vi "PicoScope4000aExampleStreaming without queue220623.vi"() -> ()   [LabVIEW 2024]
uses:
  Global variables/Global 1.vi
  Global variables/filepath global variable.vi
  Global variables/global for picoscope.vi
  LabVIEW3D/PicoScope/Pico Technology/SDK/lib/ps4000a.dll
panel:
  out "result 2":dbl
  out "size (in bytes)":i64
  out "sampling period [s]":dbl=4.0000000000000003e-07
  in  ".pico filepath":path=path "F:/20240321-194116tdTomato/waveforms.pico"
  out "result":bool=TRUE
  out "record":bool=TRUE
  in  "start":bool
  in  "Channel settings":T1={"Ch D  sync"={"Enabled"=FALSE, "Coupling"=1, "Range"=7, "Offset"=0.0}, "Ch C AWG "={"Enabled"=TRUE, "Coupling"=1, "Range"=6, "Offset"=0.0}, "Ch G scape"={"Enabled"=TRUE, "Coupling"=1, "Range"=5, " Offset"=0.0}, "Ch H img scan"={"Enabled"=TRUE, "Coupling"=1, "Range"=7, "Offset"=0.0}, "Ch B Cam"={"Enabled"=TRUE, "Coupling"=1, "Range"=9, "Offset"=0.0}, "Ch A"={"Enabled"=FALSE, "Coupling"=1, "Range"=9, "Offset"=0.0}, "Ch E"={"Enabled"=FALSE, "Coupling"=1, "Range"=2, "Offset"=0.0}, "Ch F"={"Enabled"=FALSE, "Coupling"=1, "Range"=9, "Offset"=0.0}} {"Ch F"."Range" items=["10 mV", "20 mV", "50 mV", "100 mV", "200 mV", "500 mV", "1 V", "2 V", "5 V", "10 V", "20 V", "50 V ", "100 V"]; "Ch F"."Coupling" items=["AC", "DC"]; "Ch E"."Range" items=["10 mV", "20 mV", "50 mV", "100 mV", "200 mV", "500 mV", "1 V", "2 V", "5 V", "10 V", "20 V", "50 V ", "100 V"]; "Ch E"."Coupling" items=["AC", "DC"]; "Ch A"."Range" items=["10 mV", "20 mV", "50 mV", "100 mV", "200 mV", "500 mV", "1 V", "2 V", "5 V", "10 V", "20 V", "50 V ", "100 V"]; "Ch A"."Coupling" items=["AC", "DC"]; "Ch B Cam"."Range" items=["10 mV", "20 mV", "50 mV", "100 mV", "200 mV", "500 mV", "1 V", "2 V", "5 V", "10 V", "20 V", "50 V ", "100 V"]; "Ch B Cam"."Coupling" items=["AC", "DC"]; "Ch H img scan"."Range" items=["10 mV", "20 mV", "50 mV", "100 mV", "200 mV", "500 mV", "1 V", "2 V", "5 V", "10 V", "20 V", "50 V ", "100 V"]; "Ch H img scan"."Coupling" items=["AC", "DC"]; "Ch G scape"."Range" items=["10 mV", "20 mV", "50 mV", "100 mV", "200 mV", "500 mV", "1 V", "2 V", "5 V", "10 V", "20 V", "50 V ", "100 V"]; "Ch G scape"."Coupling" items=["AC", "DC"]; "Ch C AWG"."Range" items=["10 mV", "20 mV", "50 mV", "100 mV", "200 mV", "500 mV", "1 V", "2 V", "5 V", "10 V", "20 V", "50 V ", "100 V"]; "Ch C AWG"."Coupling" items=["AC", "DC"]; "Ch D  sync"."Range" items=["10 mV", "20 mV", "50 mV", "100 mV", "200 mV", "500 mV", "1 V", "2 V", "5 V", "10 V", "20 V", "50 V ", "100 V"]; "Ch D  sync"."Coupling" items=["AC", "DC"]}
  out "Numeric":i32=2767
  in  "Trigger Settings":T2={"Trigger Enabled"=FALSE, "Trigger Source"=enum."Channel D", "Trig Thresh (16-bit counts)"=16384, "Trigger Direction"=2, "Trigger Delay (samples)"=0, "Auto Trigger Time (ms)"=0} {"Trigger Direction" items=["Rising"=2, "Falling"=3]}
  out "Triggered":bool
  out "Sample Interval":u32=200
  in  "Acquisition Settings":T3={"Auto Stop"=FALSE, "Desired Sample Interval"=200, "Pre-trigger Samples"=0, "Post-trigger Samples"=1000000, "Down-Sample Ratio"=1, "Down-Sample Mode"=0, "Overview Buffer Size"=1000000, "Time Units"=2} {"Time Units" items=["Nanoseconds (ns)"=2, "Microseconds (us)"=3, "Milliseconds (ms)"=4, "Seconds (s)"=5]; "Down-Sample Mode" items=["None"=0, "Aggregate"=1, "Decimate"=2, "Average"=4]}
  out "Total Samples":u32=172949504
  out "Auto Stopped":bool
  out "# of Smpls per Capture":u32=65536
  in  "stop":bool
  # "sampling period = time units * interval\nrecording points = pre- + post- smpls (しかしauto stop押さなければ繰り返し測定。Trigger disabled にしておくと連続測定。dead timeがどのくらいあるかは不明\n\nとりあえず全部波形保存しておけば、それで画像の時刻と同期がとれるので問題なし。"
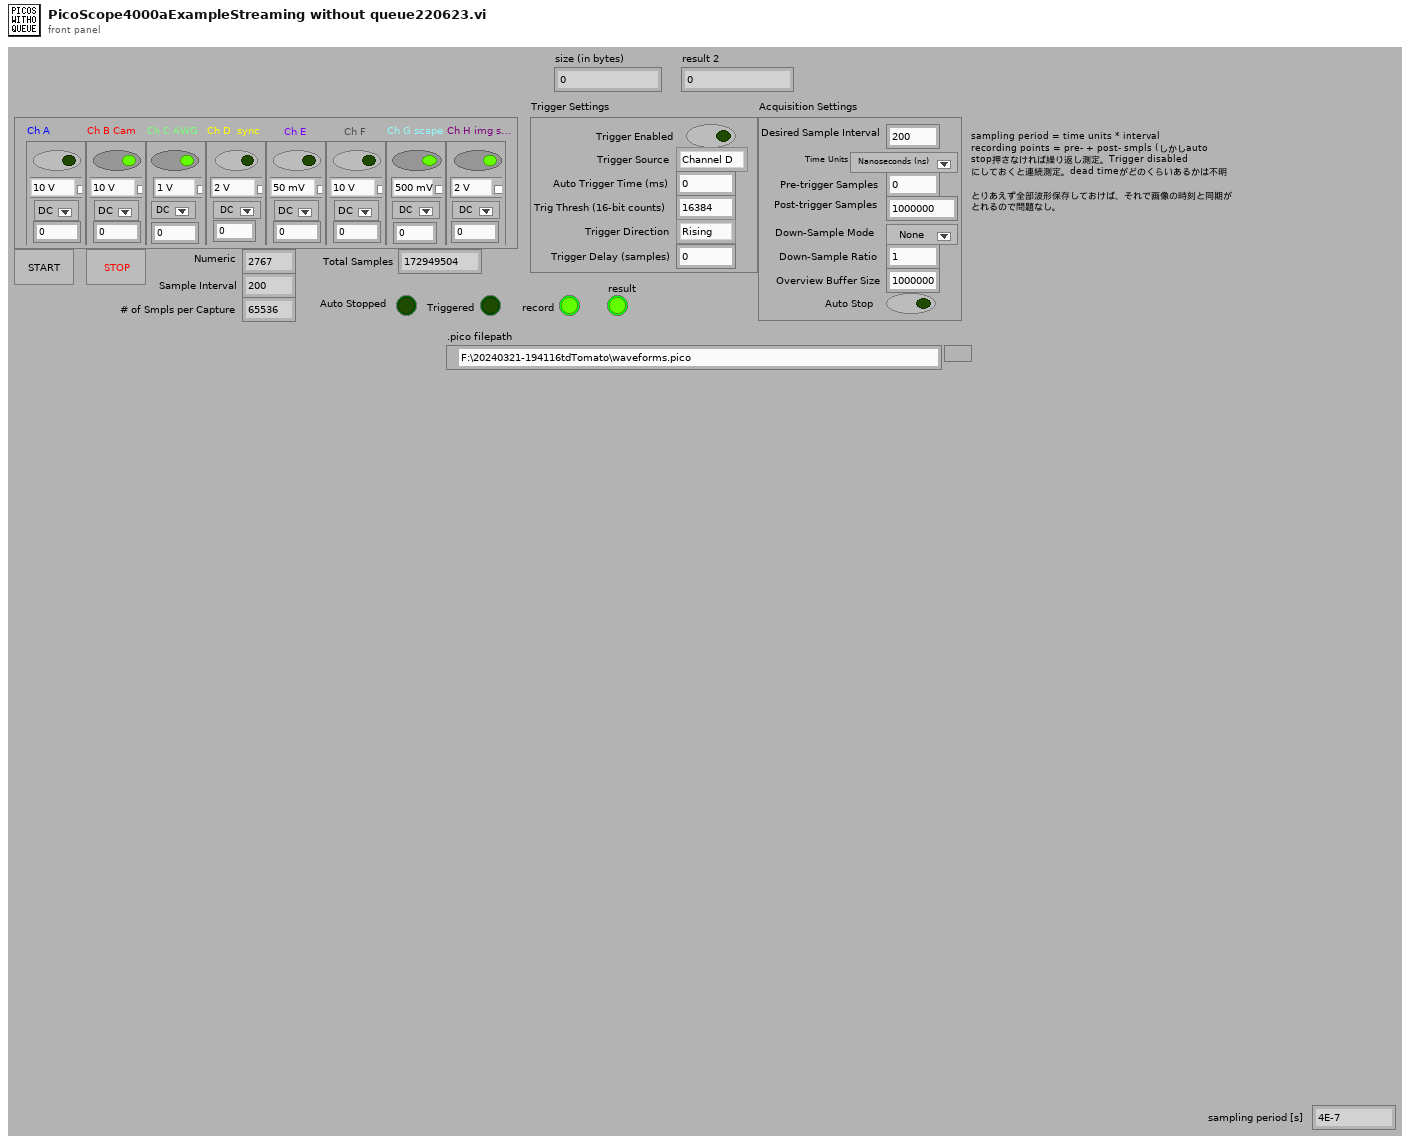
[diagram p1: front panel]
types:
  T1 = cluster{"Ch D  sync":cluster{"Enabled":bool, "Coupling":i16, "Range":u16, "Offset":sgl}, "Ch C AWG ":cluster{"Enabled":bool, "Coupling":i16, "Range":u16, "Offset":sgl}, "Ch G scape":cluster{"Enabled":bool, "Coupling":i16, "Range":u16, " Offset":sgl}, "Ch H img scan":cluster{"Enabled":bool, "Coupling":i16, "Range":u16, "Offset":sgl}, "Ch B Cam":cluster{"Enabled":bool, "Coupling":i16, "Range":u16, "Offset":sgl}, "Ch A":cluster{"Enabled":bool, "Coupling":i16, "Range":u16, "Offset":sgl}, "Ch E":cluster{"Enabled":bool, "Coupling":i16, "Range":u16, "Offset":sgl}, "Ch F":cluster{"Enabled":bool, "Coupling":i16, "Range":u16, "Offset":sgl}}
  T2 = cluster{"Trigger Enabled":bool, "Trigger Source":enum16{"Channel A", "Channel B", "Channel C", "Channel D", "Channel E", "Channel F", "Channel G", "Channel H"}, "Trig Thresh (16-bit counts)":i16, "Trigger Direction":u16, "Trigger Delay (samples)":u32, "Auto Trigger Time (ms)":i16}
  T3 = cluster{"Auto Stop":bool, "Desired Sample Interval":u32, "Pre-trigger Samples":u32, "Post-trigger Samples":u32, "Down-Sample Ratio":u32, "Down-Sample Mode":i32, "Overview Buffer Size":u32, "Time Units":u32}
  T4 = cluster{"Channel settings":cluster{"Ch D  sync":cluster{"Enabled":bool, "Coupling":i16, "Range":u16, "Offset":sgl}, "Ch C AWG ":cluster{"Enabled":bool, "Coupling":i16, "Range":u16, "Offset":sgl}, "Ch G scape":cluster{"Enabled":bool, "Coupling":i16, "Range":u16, " Offset":sgl}, "Ch H img scan":cluster{"Enabled":bool, "Coupling":i16, "Range":u16, "Offset":sgl}, "Ch B Cam":cluster{"Enabled":bool, "Coupling":i16, "Range":u16, "Offset":sgl}, "Ch A":cluster{"Enabled":bool, "Coupling":i16, "Range":u16, "Offset":sgl}, "Ch E":cluster{"Enabled":bool, "Coupling":i16, "Range":u16, "Offset":sgl}, "Ch F":cluster{"Enabled":bool, "Coupling":i16, "Range":u16, "Offset":sgl}}, "Acquisition Settings":cluster{"Auto Stop":bool, "Desired Sample Interval":u32, "Pre-trigger Samples":u32, "Post-trigger Samples":u32, "Down-Sample Ratio":u32, "Down-Sample Mode":i32, "Overview Buffer Size":u32, "Time Units":u32}, "Trigger Settings":cluster{"Trigger Enabled":bool, "Trigger Source":enum16{"Channel A", "Channel B", "Channel C", "Channel D", "Channel E", "Channel F", "Channel G", "Channel H"}, "Trig Thresh (16-bit counts)":i16, "Trigger Direction":u16, "Trigger Delay (samples)":u32, "Auto Trigger Time (ms)":i16}}
  T5 = enum16{"open", "replace", "create", "open or create", "replace or create", "replace or create with confirmation"}
  T6 = cluster{"Driver Version":string, "USB Version":string, "Hardware":string, "Variant":string, "Batch and Serial":string, "Cal Date":string, "Kernel Version":string, "Digital HW Version":string, "Analogue HW Version":string, "Firmware 1":string, "Firmware 2":string, "Num. channels":i16}
  T7 = cluster{"Enabled":bool, "Coupling":i16, "Range":u16, "Offset":sgl}
  T8 = cluster{"Enabled":bool, "Coupling":i16, "Range":u16, " Offset":sgl}
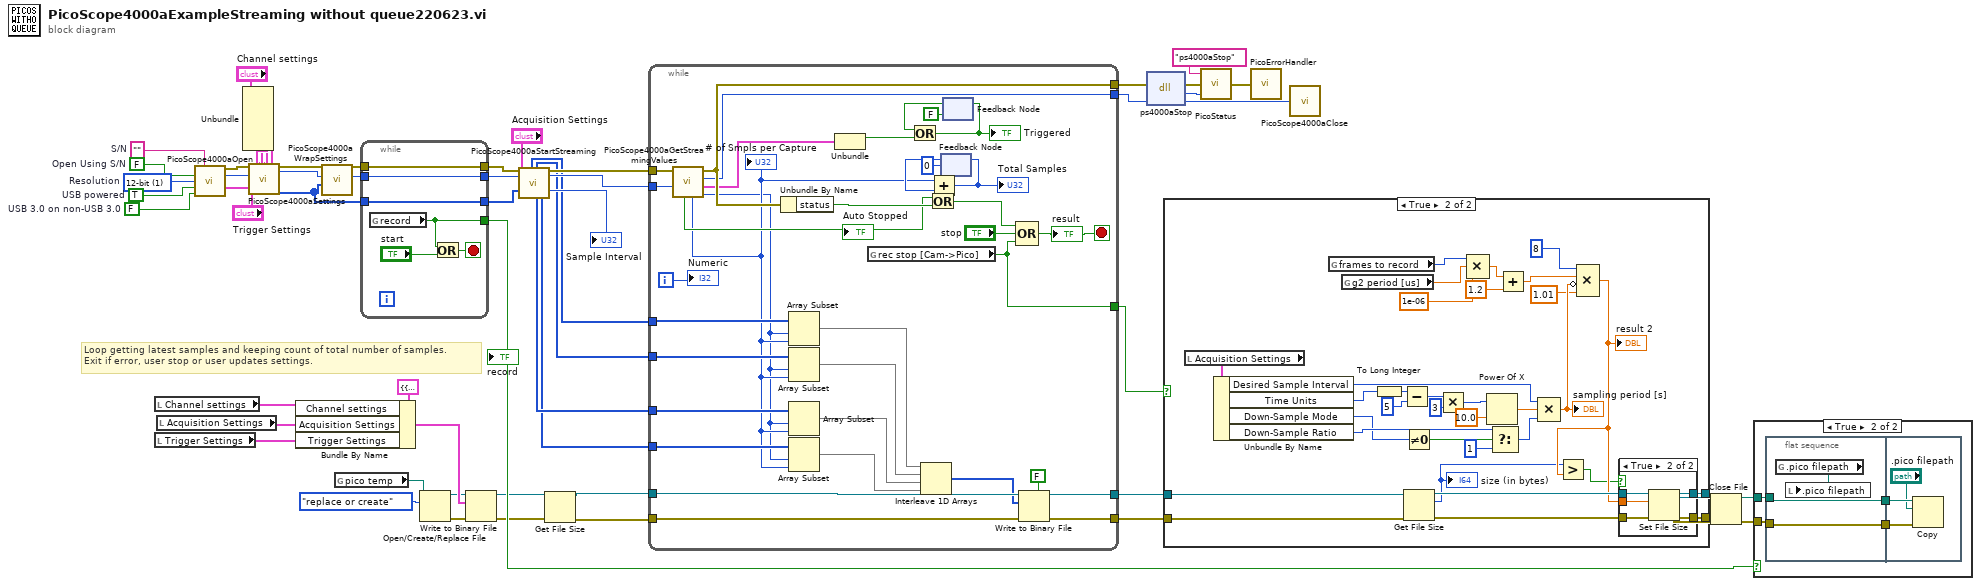
[diagram p0: block diagram]
diagram:
  w59 = ""  # S/N
  w60 = FALSE  # Open Using S/N
  w54 = u16 1 items=["12-bit"=1, "14-bit"=2]  # Resolution
  w56 = FALSE  # USB 3.0 on non-USB 3.0
  w57 = TRUE  # USB powered
  # "Loop getting latest samples and keeping count of total number of samples. \nExit if error, user stop or user updates settings."
  n1 = local read "Channel settings"() -> (w21:T1)
  n2 = local read "Trigger Settings"() -> (w20:T2)
  n3 = local read "Acquisition Settings"() -> (w19:T3)
  n4 = call "PicoScope4000aOpen.vi"("Serial Number"=w59, "Use Serial Number"=w60, "Resolution"=w54, "USB powered control"=w57, "USB 3.0 on non-USB 3.0 port control"=w56) -> ("error out"=w62:errorcluster, "handle"=w61:i16, "Unit Info"=w55:T6)  [unwired: 5 in, 3 out]
  n5 = Unbundle("Channel settings") -> ("Ch D  sync"=w38:T7, "Ch C AWG"=w37:T7, "Ch G scape"=w36:T8, "Ch H img scan"=w35:T7, "Ch B Cam"=w39:T7, "Ch A"=w40:T7, "Ch E"=w34:T7, "Ch F"=w33:T7)
  n6 = call "PicoScope4000aSettings.vi"("error in"=w62, "handle in"=w61, "Trigger Settings"="Trigger Settings", "Channel A Settings"=w40, "Channel E Settings"=w34, "Channel B Settings"=w39, "Channel F Settings"=w33, "Channel C Settings"=w37, "Channel G Settings"=w36, "Channel D Settings"=w38, "Channel H Settings"=w35, "Unit Info"=w55) -> ("error out"=w47:errorcluster, "handle out"=w46:i16, "Enabled array"=w25:i16[])  [unwired: 5 in]
  n7 = Bundle By Name(cluster=T4 {"Channel settings"={"Ch D  sync"={"Enabled"=FALSE, "Coupling"=0, "Range"=0, "Offset"=0.0}, "Ch C AWG "={"Enabled"=FALSE, "Coupling"=0, "Range"=0, "Offset"=0.0}, "Ch G scape"={"Enabled"=FALSE, "Coupling"=0, "Range"=0, " Offset"=0.0}, "Ch H img scan"={"Enabled"=FALSE, "Coupling"=0, "Range"=0, "Offset"=0.0}, "Ch B Cam"={"Enabled"=FALSE, "Coupling"=0, "Range"=0, "Offset"=0.0}, "Ch A"={"Enabled"=FALSE, "Coupling"=0, "Range"=0, "Offset"=0.0}, "Ch E"={"Enabled"=FALSE, "Coupling"=0, "Range"=0, "Offset"=0.0}, "Ch F"={"Enabled"=FALSE, "Coupling"=0, "Range"=0, "Offset"=0.0}}, "Acquisition Settings"={"Auto Stop"=FALSE, "Desired Sample Interval"=0, "Pre-trigger Samples"=0, "Post-trigger Samples"=0, "Down-Sample Ratio"=0, "Down-Sample Mode"=0, "Overview Buffer Size"=0, "Time Units"=0}, "Trigger Settings"={"Trigger Enabled"=FALSE, "Trigger Source"=enum."Channel A", "Trig Thresh (16-bit counts)"=0, "Trigger Direction"=0, "Trigger Delay (samples)"=0, "Auto Trigger Time (ms)"=0}} ("output cluster"), "Channel settings"=w21, "Acquisition Settings"=w19, "Trigger Settings"=w20) -> (w17:T4)
  n8 = call "PicoScope4000aWrapSettings.vi"("Enabled array"=w25, "Handle In"=w46, "error in (no error)"=w47) -> ("Handle Out"=w26:i16, "error out"=w27:errorcluster)  [unwired: 7 in]
  n9 = global read "filepath global variable.vi" "pico temp"() -> (w1:path)
  n10 = while {
    tunnel: w27 -> [w68]
    tunnel: w26 -> [w67]
    tunnel: w25 -> [w66]
    tunnel: [w68] -> w24
    tunnel: [w67] -> w23
    tunnel: [w66] -> w22
    tunnel: [w63] -> w11
    stop <- w65 stop-if-true
    n11 = global read "Global 1.vi" "record"() -> (w63:bool)
    n12 = Or(x=w63, y="start") -> (x .or. y?=w65:bool)
  }
  "record" <- w11
  n13 = Open/Create/Replace File(file path (use dialog)=w1, operation (0:open)=T5."replace or create") -> (refnum out=w16:refnum<file>, error out=w15:errorcluster)  [unwired: 4 in, 1 out]
  n14 = Write to Binary File(file (use dialog)=w16, data=w17, error in=w15) -> (refnum out=w10:refnum<file>, error out=w9:errorcluster)  [unwired: 3 in, 1 out]
  n15 = call "PicoScope4000aStartStreaming.vi"("error in"=w24, "handle in"=w23, "Enabled array"=w22, "Acquisition Settings"="Acquisition Settings") -> ("Channel B"=w30:i16[], "Channel C"=w29:i16[], "Channel G"=w32:i16[], "Channel H"=w28:i16[], "error out"=w31:errorcluster, "handle out"=w45:i16, "Sample Interval"=→"Sample Interval":u32)  [unwired: 5 in, 4 out]
  n16 = Get File Size(file=w10, error in=w9) -> (refnum out=w8:refnum<file>, 0:w7:errorcluster)  [unwired: 1 out]
  n17 = while {
    tunnel: [w91] -> w53
    tunnel: w45 -> [w93]
    tunnel: w31 -> [w94]
    tunnel: [w92] -> w52
    tunnel: w32 -> [w87]
    tunnel: w30 -> [w83]
    tunnel: w29 -> [w84]
    tunnel: w28 -> [w85]
    tunnel: w7 -> [w74]
    tunnel: w8 -> [w73]
    tunnel: [w72] -> w6
    tunnel: [w71] -> w3
    tunnel: [w69] -> w2
    i -> [w88]
    stop <- w77 stop-if-true
    n18 = call "PicoScope4000aGetStreamingValues.vi"("handle in"=w93, "error in"=w94) -> ("Start Index in Driver Buffer"=w81:u32, "Trigger"=w90:cluster{bool, "triggeredAt (Total samples)":u32}, "handle out"=w91:i16, "error out"=w92:errorcluster, "Number of Samples"=w82:u32, "Auto Stopped"=w89:bool)  [unwired: 4 in]
    "Auto Stopped" <- w89
    "# of Smpls per Capture" <- w82
    n19 = Unbundle By Name(w92) -> ("status"=w102:bool)
    n20 = Array Subset(array=w83, index=w81, length=w82) -> (w76:i16[])
    n21 = Array Subset(array=w84, index=w81, length=w82) -> (w80:i16[])
    n22 = Array Subset(array=w87, index=w81, length=w82) -> (w79:i16[])
    n23 = Array Subset(array=w85, index=w81, length=w82) -> (w78:i16[])
    n24 = Unbundle(w90) -> (w96:bool)  [unwired: 1 out]
    n25 = global read "Global 1.vi" "rec stop [Cam->Pico]"() -> (w69:bool)
    n26 = Interleave 1D Arrays(w76, w80, w79, w78) -> (w70:i16[])
    n27 = Or(x=w89, y=w102) -> (x .or. y?=w101:bool)
    n28 = feedback #1(u32 0) -> (w95:u32)
    n29 = Add(x=w82, y=w95) -> (x+y=w99:u32)
    "Total Samples" <- w99
    n30 = feedback-in #1(w99) -> ()
    n31 = feedback #2(FALSE) -> (w98:bool)
    n32 = Or(x=w98, y=w96) -> (x .or. y?=w86:bool)
    "Triggered" <- w86
    n33 = feedback-in #2(w86) -> ()
    n34 = Compound Arithmetic op=OR(w101, "stop", w69) -> (w77:bool)
    "result" <- w77
    n35 = Write to Binary File(file (use dialog)=w73, data=w70, error in=w74, 5:FALSE ("prepend array or string size? (T)")) -> (refnum out=w71:refnum<file>, error out=w72:errorcluster)  [unwired: 2 in, 1 out]
    "Numeric" <- w88
  }
  n36 = dll-call lib="C:/Users/Mikamilab/Documents/lightsheet/LabVIEW3D/PicoScope/Pico Technology/SDK/lib/ps4000A.dll" fn="ps4000aStop"(error in=w52, "handle"=w53) -> (error out=w50:errorcluster, "PICO_STATUS"=w51:u32, "handle"=w58:i16)  [unwired: 2 in, 1 out]
  n37 = case shown="True" w2 {
    tunnel: w6 -> [w104 w120]
    tunnel: [w104 w118] -> w5
    tunnel: [w105 w117] -> w4
    tunnel: w3 -> [w105 w116]
    frame False {
    }
    frame True {
      n38 = local read "Acquisition Settings"() -> (w124:T3)
      n39 = Unbundle By Name(w124) -> ("Desired Sample Interval"=w131:u32, "Time Units"=w125:u32, "Down-Sample Mode"=w133:i32, "Down-Sample Ratio"=w135:u32)
      n40 = global read "global for picoscope.vi" "frames to record"() -> (w114:i32)
      n41 = global read "global for picoscope.vi" "g2 period [us]"() -> (w113:dbl)
      n42 = To Long Integer(number=w125) -> (32bit integer=w138:i32)
      n43 = Subtract(x=w138, y=5 ("x")) -> (x-y=w127:i32)
      n44 = Not Equal To 0?(x=w133) -> (x != 0?=w134:bool)
      n45 = Get File Size(file=w116, error in=w120) -> (refnum out=w115:refnum<file>, size (in bytes)=w107:i64, 0:w119:errorcluster)
      "size (in bytes)" <- w107
      n46 = Multiply(x=w127, y=3) -> (x*y=w130:i32)
      n47 = Compound Arithmetic op=MULTIPLY(w114, w113, 1e-06 ("value")) -> (w111:dbl)
      n48 = Power Of X(1:10.0 ("x"), 2:w130) -> (0:w132:dbl)
      n49 = Select(t=w135, s=w134, f=1) -> (s? t:f=w137:u32)
      n50 = Add(x=w111, y=1.2) -> (x+y=w109:dbl)
      n51 = Compound Arithmetic op=MULTIPLY(w131, w132, w137) -> (w123:dbl)
      "sampling period [s]" <- w123
      n52 = Compound Arithmetic op=MULTIPLY(8 ("value"), w109, invert w123, 1.01 ("value")) -> (w108:dbl)
      "result 2" <- w108
      n53 = Greater?(x=w107, y=w108) -> (0:w106:bool)
      n54 = case shown="True" w106 {
        tunnel: w119 -> [w139 w145]
        tunnel: [w139 w144] -> w118
        tunnel: [w140 w143] -> w117
        tunnel: w115 -> [w140 w142]
        tunnel: w108 -> [_ w141]
        frame False {
        }
        frame True {
          n55 = Set File Size(4:w145, 6:w141, 7:w142) -> (0:w144:errorcluster, 3:w143:refnum<file>)
        }
      }
    }
  }
  n56 = call "PicoStatus.vi"("PICO STATUS"=w51, "error in"=w50, "source"="ps4000aStop") -> ("error out"=w49:errorcluster)
  n57 = call "PicoErrorHandler.vi"("error in"=w49) -> ()  [unwired: 1 out]
  n58 = call "PicoScope4000aClose.vi"("handle"=w58) -> ()
  n59 = Close File(refnum=w4, error in=w5) -> (path=w12:path, error out=w13:errorcluster)
  n60 = case shown="True" w11 {
    tunnel: w13 -> [_ w147]
    tunnel: w12 -> [_ w146]
    frame False {
    }
    frame True {
      n61 = flat-sequence {
        tunnel: w146 -> [w152]
        tunnel: w147 -> [w151]
        tunnel: [w152] -> w149
        tunnel: [w151] -> w148
        tunnel: w149 -> [w155]
        tunnel: w148 -> [w154]
        frame #0 {
          n62 = global read "Global 1.vi" ".pico filepath"() -> (w150:path)
          n63 = local write ".pico filepath"(w150) -> ()
        }
        frame #1 {
          n64 = Copy(8:w154, 10:".pico filepath", 11:w155) -> ()  [unwired: 2 in, 3 out]
        }
      }
    }
  }
